vi "Read Page Size.vi"(0 "PDF Report":T21(xcontrol), 11 "error in (no error)":errorcluster) -> (4 "PDF Report duplicate":T21(xcontrol), 6 "Text zone (points)":cluster{"widht":sgl, "height":sgl}={"widht"=612.0, "height"=792.0}, 10 "Page (points)":T1={"Start at page"=1, "Orientation"=enum."Portrait", "widht"=612.0, "height"=792.0, "Margin left"=72.0, "Margin right"=72.0, "Margin top"=72.0, "Margin bottom"=72.0}, 15 "error out":errorcluster)   [LabVIEW 2012]
doc: "Version 1.0\nDeveloped by Jean-Marc Simard\nCopyright © 2010, Exaprom Inc.\nAll rights reserved.\nLicense: BSD\n\nWith iTextSharp 4.1.6 (http://itextsharp.sourceforge.net)\nunder Mozilla Public License Version 1.1\n(http://www.mozilla.org/MPL/MPL-1.1.html)"
uses:
  Controls/PDF Report Xcontrol/PDF Report.xctl
  Controls/Page dimensions.ctl
  Controls/Page Orientation.ctl
  C:/Users/MaxCorp/Documents/TopPerm - Base/DLL/itextsharp.dll
  DLL/itextsharp.dll
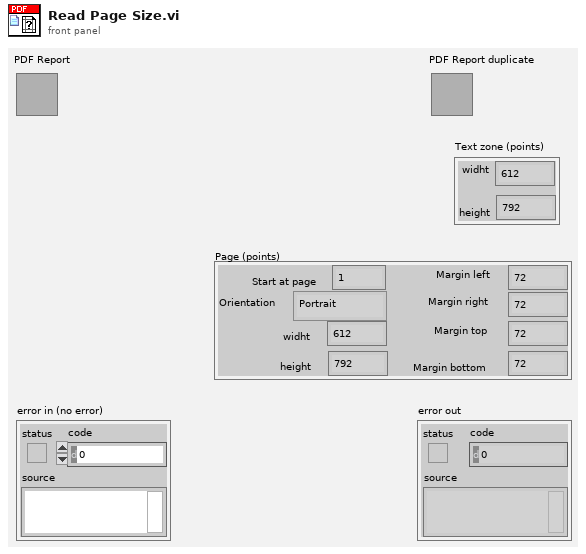
[diagram p1: front panel]
types:
  T1 = typedef "Page dimensions.ctl" = cluster{"Start at page":i32, "Orientation":T2, "widht":sgl, "height":sgl, "Margin left":sgl, "Margin right":sgl, "Margin top":sgl, "Margin bottom":sgl}
  T2 = typedef "Page Orientation.ctl" = enum16{"Portrait", "Landscape"}
  T3 = typedef "Font cluster.ctl" = cluster{"Name":string, "Size":T4, "Color":T5, "Style":cluster{"Bold":bool, "Italic":bool, "Underline":bool, "Strikeout":bool}}
  T4 = typedef "Font size.ctl" = sgl
  T5 = typedef "Font color.ctl" = u32
  T6 = typedef "Unit.ctl" = enum16{"inch", "mm"}
  T7 = typedef "Paragraphe cluster.ctl" = cluster{" Aligment":T8, "Line spacing":T9}
  T8 = typedef "Texte alignement.ctl" = enum16{"Select", "CENTER", "JUSTIFY", "LEFT", "RIGHT"}
  T9 = typedef "Line spacing.ctl" = enum16{"Select", "1.0", "1.5", "2.0"}
  T10 = typedef "Image or Table Caption.ctl" = cluster{"Caption":string, "Separator":string, "Position":enum16{"Above", "Below"}}
  T11 = typedef "Header Footer [ ].ctl" = T12[]
  T12 = typedef "Header Footer cluster.ctl" = cluster{"Start page":i32, "Type":T13, "Alignment":T14, "Vertical Alignement":T15, "Image (%)":sgl, "Page #":T16, "Text":string, "Path":string, "Font":T3, "Font refnum":refnum<k24>, "Line":cluster{"Line":T17, "Thickness (points)":sgl, "Colour":T5}}
  T13 = typedef "Header Footer Type.ctl" = enum16{"Select", "Text", "Text + hyperlink", "Page number", "Image", "Image + hyperlink"}
  T14 = typedef "Header footer horiz alignment.ctl" = enum16{"Left", "Center", "Right"}
  T15 = typedef "Cell Vertical alignment.ctl" = enum16{"TOP", "MIDDLE", "BOTTOM"}
  T16 = typedef "Page number.ctl" = cluster{"Text 1":string, "Text 2":string, "Text 3":string}
  T17 = typedef "Header Footer Line.ctl" = enum16{"No line", "Horizontal line"}
  T18 = typedef "Watermark cluster2.ctl" = cluster{"Show? (F)":bool, "Type":enum16{"Image", "Text"}, "Opacity (%)":sgl, "Rotate(°)":sgl, "Position":cluster{"Position":T19, "X":sgl, "Y":sgl}, "Image path":path, "Scaled(%)":sgl, "Image refnum":refnum<k24>, "Text":string, "Font":cluster{"Name":string, "Size":T4, "Color":T5}, "Font refnum":refnum<k24>, "Alignment":T14, "Automatic":bool}
  T19 = typedef "Watermark Position.ctl" = enum16{"Absolute", "Center (page)", "Center (text section)"}
  T20 = typedef "System Fonts.ctl" = cluster{"Font name [ ]":string[], "Font and file names [ ]":cluster{"Font name":string, "File name":string}[]}
  T21 = cluster{"Document":refnum<k24>, "Writer":refnum<k24>, "Default Font":refnum<k24>, "Default Font cluster":T3, "Path":path, "Unit (default = mm)":T6, "Paragraphe cluster":T7, "Pages dimensions [ ]":T1[], "Captions":cluster{"Image":T10, "Image counter":u16, "Table":T10, "Table counter":u16, "Font":T3}, "Header":T11, "Footer":T11, "Watermark ":T18, "Actual VI name":string, "System Fonts":T20}
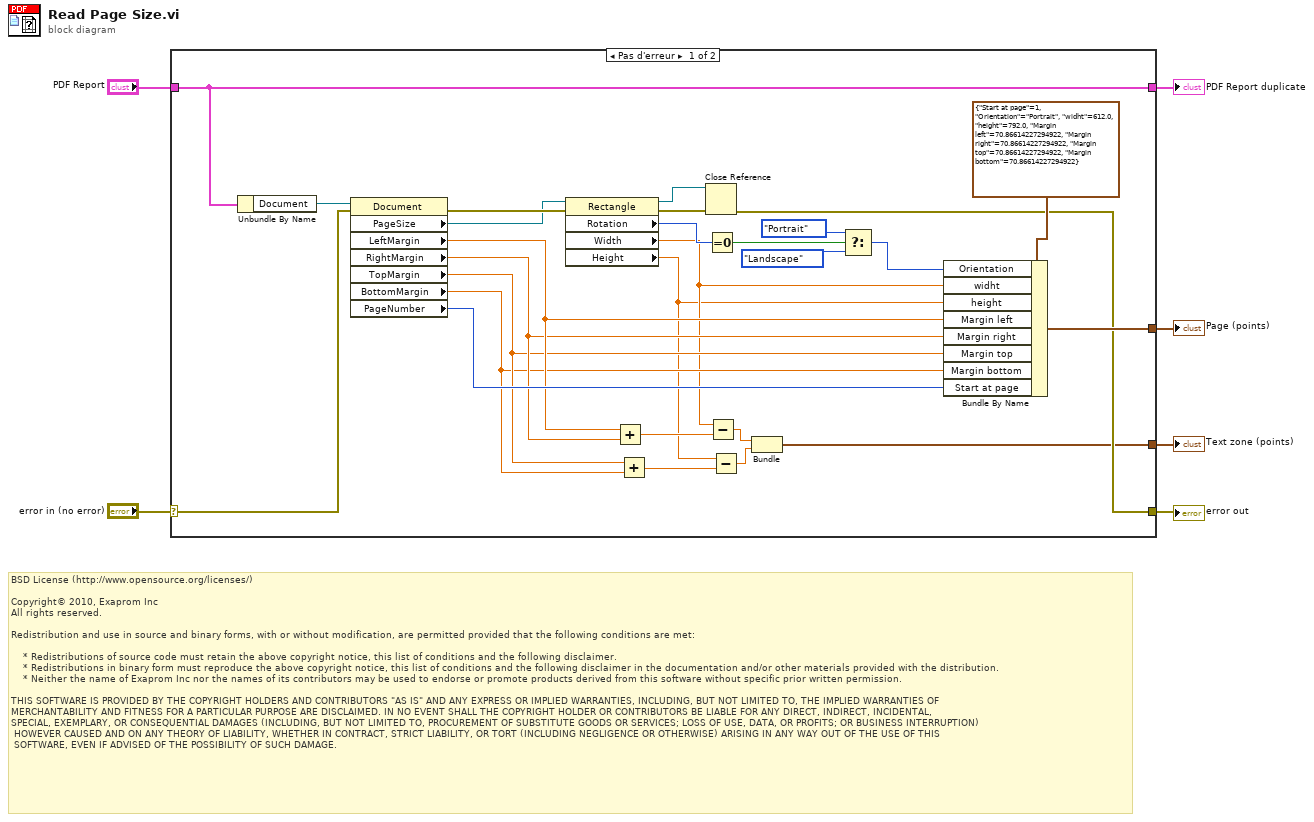
[diagram p0: block diagram]
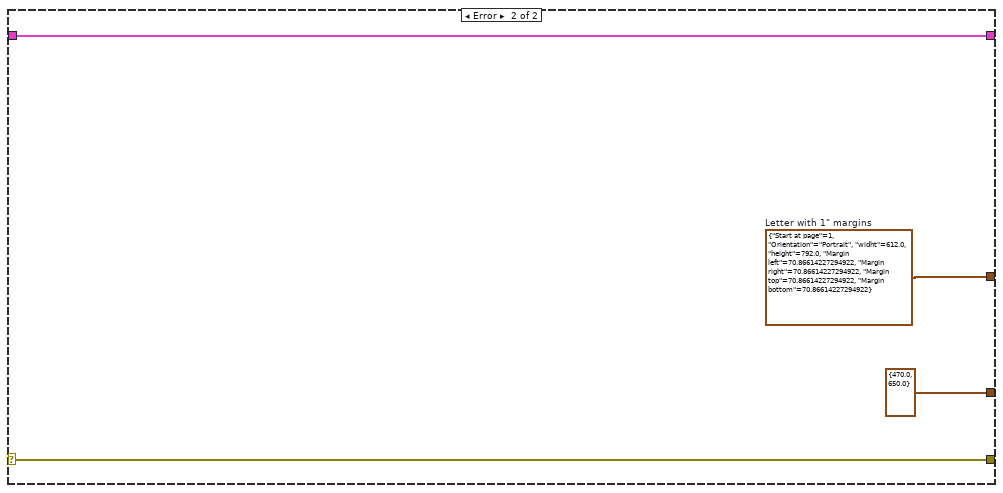
[diagram p2: hidden frame]
diagram:
  # "BSD License (http://www.opensource.org/licenses/)\n\nCopyright© 2010, Exaprom Inc\nAll rights reserved.\n\nRedistribution and use in source and binary forms, with or without modification, are permitted provided that the following conditions are met:\n\n    * Redistributions of source code must retain the above copyright notice, this list of conditions and the following disclaimer.\n    * Redistributions in binary form must reproduce the above copyright notice, this list of conditions and the following disclaimer in the documentation and/or other materials provided with the distribution.\n    * Neither the name of Exaprom Inc nor the names of its contributors may be used to endorse or promote products derived from this software without specific prior written permission.\n\nTHIS SOFTWARE IS PROVIDED BY THE COPYRIGHT HOLDERS AND CONTRIBUTORS \"AS IS\" AND ANY EXPRESS OR IMPLIED WARRANTIES, INCLUDING, BUT NOT LIMITED TO, THE IMPLIED WARRANTIES OF \nMERCHANTABILITY AND FITNESS FOR A PARTICULAR PURPOSE ARE DISCLAIMED. IN NO EVENT SHALL THE COPYRIGHT HOLDER OR CONTRIBUTORS BE LIABLE FOR ANY DIRECT, INDIRECT, INCIDENTAL,\nSPECIAL, EXEMPLARY, OR CONSEQUENTIAL DAMAGES (INCLUDING, BUT NOT LIMITED TO, PROCUREMENT OF SUBSTITUTE GOODS OR SERVICES; LOSS OF USE, DATA, OR PROFITS; OR BUSINESS INTERRUPTION)\n HOWEVER CAUSED AND ON ANY THEORY OF LIABILITY, WHETHER IN CONTRACT, STRICT LIABILITY, OR TORT (INCLUDING NEGLIGENCE OR OTHERWISE) ARISING IN ANY WAY OUT OF THE USE OF THIS\n SOFTWARE, EVEN IF ADVISED OF THE POSSIBILITY OF SUCH DAMAGE."
  n1 = case shown="Pas d'erreur" "error in (no error)" {
    selector: "error in (no error)" -> [w19 w37]
    tunnel: [w27 w35] -> w6
    tunnel: "PDF Report" -> [w22 w36]
    tunnel: [w18 w37] -> w3
    tunnel: [w22 w36] -> w2
    tunnel: [w7 cluster{sgl, sgl} {470.0, 650.0}] -> w1
    frame No Error {
      n2 = Unbundle By Name(w22) -> ("Document"=w24:refnum<k24>)
      n3 = property class="Document"(reference=w24, error in=w19) -> (error out=w33:errorcluster, "PageSize"=w32:refnum<k24>, "LeftMargin"=w17:sgl, "RightMargin"=w16:sgl, "TopMargin"=w15:sgl, "BottomMargin"=w14:sgl, "PageNumber"=w23:i32)  [unwired: 1 out]
      n4 = property class="Rectangle"(reference=w32, error in=w33) -> (reference out=w20:refnum<k24>, error out=w21:errorcluster, "Rotation"=w26:i32, "Width"=w13:sgl, "Height"=w11:sgl)
      n5 = Add(x=w17, y=w16) -> (x+y=w12:sgl)
      n6 = Add(x=w15, y=w14) -> (x+y=w10:sgl)
      n7 = Close Reference(reference=w20, error in (no error)=w21) -> (error out=w18:errorcluster)
      n8 = Equal To 0?(x=w26) -> (x = 0?=w31:bool)
      n9 = Subtract(x=w13, y=w12) -> (x-y=w9:sgl)
      n10 = Subtract(x=w11, y=w10) -> (x-y=w8:sgl)
      n11 = Bundle(w9, w8) -> (w7:cluster{sgl, sgl})  [unwired: 1 out]
      n12 = Select(t=Page_Orientation."Portrait" ("Orientation"), s=w31, f=Page_Orientation."Landscape" ("Orientation")) -> (s? t:f=w25:T2)
      n13 = Bundle By Name(cluster=T1 {"Start at page"=1, "Orientation"=enum."Portrait", "widht"=612.0, "height"=792.0, "Margin left"=70.86614, "Margin right"=70.86614, "Margin top"=70.86614, "Margin bottom"=70.86614} ("Page (points)"), "Orientation"=w25, "widht"=w13, "height"=w11, "Margin left"=w17, "Margin right"=w16, "Margin top"=w15, "Margin bottom"=w14, "Start at page"=w23) -> (w27:T1)
    }
    frame Error {
      w35 = T1 {"Start at page"=1, "Orientation"=enum."Portrait", "widht"=612.0, "height"=792.0, "Margin left"=70.86614, "Margin right"=70.86614, "Margin top"=70.86614, "Margin bottom"=70.86614}  # Letter with 1" margins
    }
  }
  "PDF Report duplicate" <- w2
  "Page (points)" <- w6
  "error out" <- w3
  "Text zone (points)" <- w1
